vi "Dyn rolling avg.vi"(2 "N":i32=3, 4 "orig array":dbl[](array[numeric])) -> (1 "moving centered avg":dbl[](array[numeric]))   [LabVIEW 2022 SP3]
uses:
  <vilib>/Analysis/baseanly.llb/Mean (DBL).vi
  <vilib>/Analysis/NI_AALBase.lvlib
panel:
  out "Gradient Theshold":dbl
  out "Max Gradient":dbl
  out "Waveform Graph":dbl[][](graph)
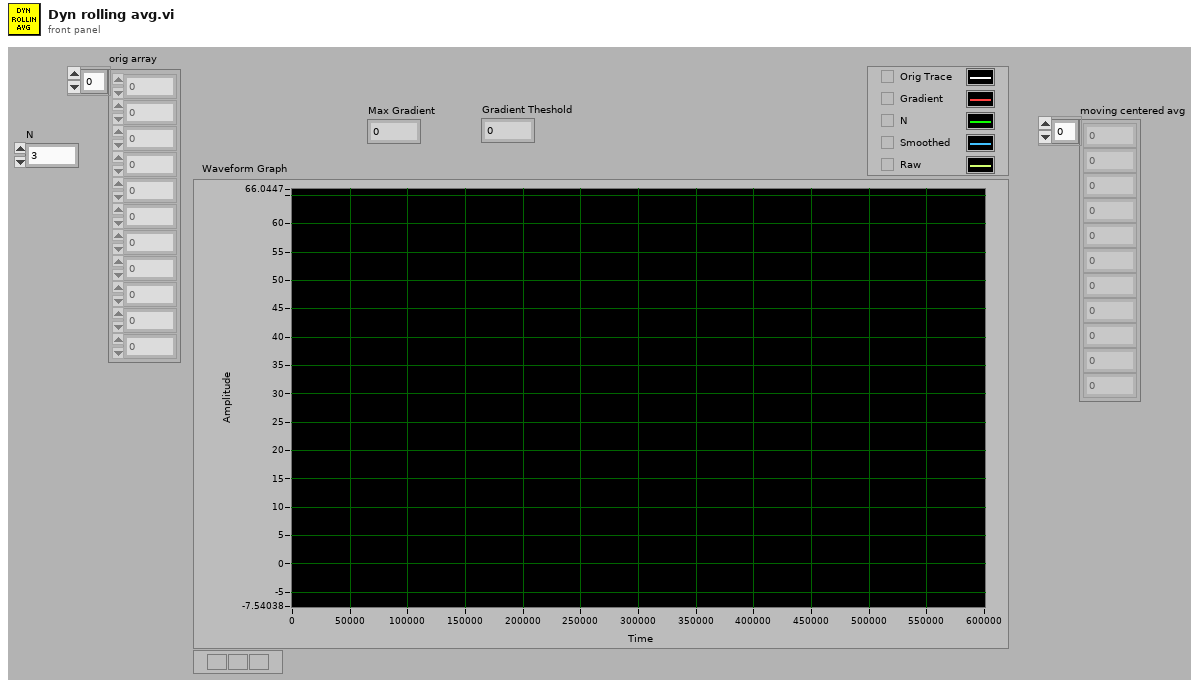
[diagram p1: front panel]
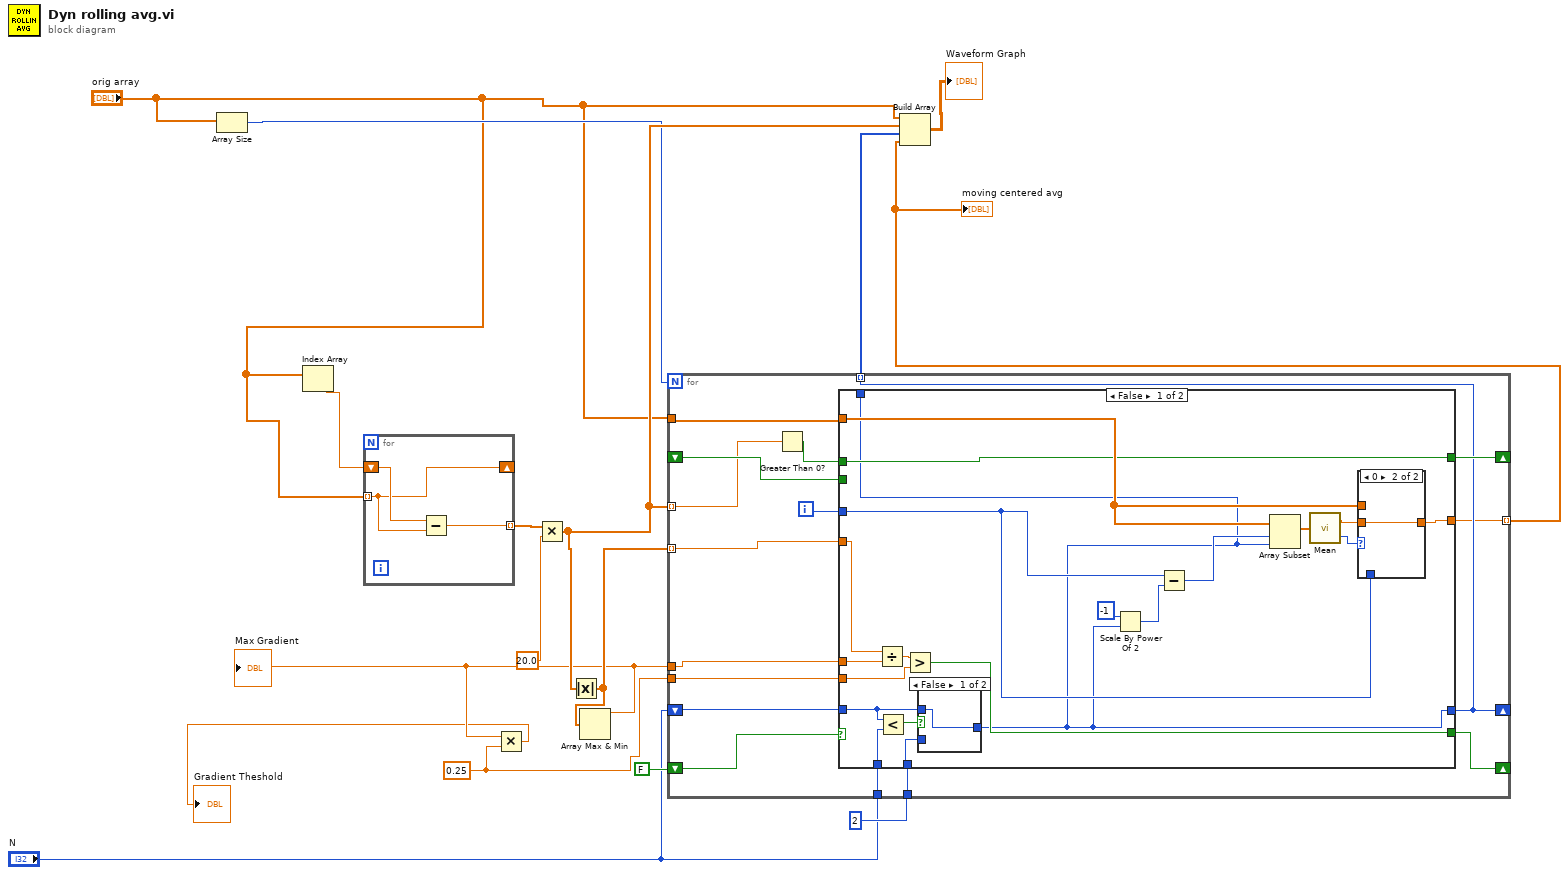
[diagram p0: block diagram]
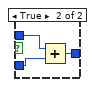
[diagram p2: hidden frame]
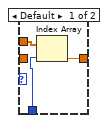
[diagram p3: hidden frame]
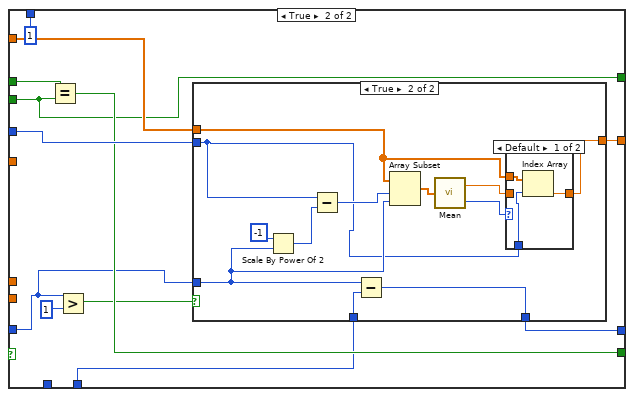
[diagram p4: hidden frame]
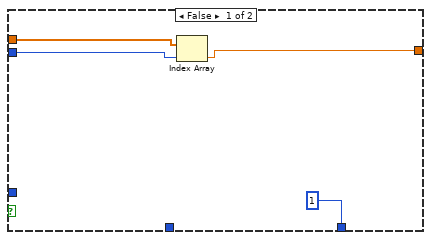
[diagram p5: hidden frame]
diagram:
  w4 = 0.25 ("y")
  n1 = Array Size(array="orig array") -> (size(s)=w7:i32)
  n2 = Index Array(array="orig array") -> (element=w15:dbl)  [unwired: 1 in]
  n3 = for {
    tunnel: "orig array" -> [w18] mode=indexing
    shift-right: [w18] -> _
    shift-left: w15 -> [w19]
    tunnel: [w17] -> w13 mode=indexing
    n4 = Subtract(x=w19, y=w18) -> (x-y=w17:dbl)
  }
  n5 = Multiply(x=w13, y=20.0) -> (x*y=w11:dbl[])
  n6 = Absolute Value(x=w11) -> (abs(x)=w12:dbl[])
  n7 = Array Max & Min(array=w12) -> (max value=w3:dbl)  [unwired: 3 out]
  "Max Gradient" <- w3
  n8 = Multiply(x=w3, y=w4) -> (x*y=→"Gradient Theshold":dbl)
  n9 = for {
    N: w7 -> [_]
    tunnel: w12 -> [w26] mode=indexing
    tunnel: w3 -> [w27]
    tunnel: "orig array" -> [w34]
    shift-right: [w31] -> _
    shift-left: _ -> [w33]
    tunnel: w11 -> [w32] mode=indexing
    shift-right: [w28] -> _
    shift-left: FALSE -> [w29]
    tunnel: [w22] -> w9 mode=indexing
    shift-right: [w22] -> _
    shift-left: "N" -> [w25]
    tunnel: 2 ("n") -> [w24]
    tunnel: "N" -> [w23]
    tunnel: w4 -> [w21]
    tunnel: [w20] -> w1 mode=indexing
    i -> [w35]
    n10 = Greater Than 0?(x=w32) -> (x > 0?=w30:bool)
    n11 = case shown="False" w29 {
      tunnel: [w55 w73] -> w20
      tunnel: w35 -> [w43 w74]
      tunnel: w34 -> [w54 w75]
      tunnel: w33 -> [_ w70]
      tunnel: [w50 w70] -> w31
      tunnel: w30 -> [w50 w72]
      tunnel: [w46 w71] -> w28
      tunnel: w27 -> [w48 _]
      tunnel: w26 -> [w47 _]
      tunnel: [w37 1 ("N")] -> _
      tunnel: w25 -> [w38 w68]
      tunnel: w24 -> [w39 w67]
      tunnel: [w37 w65] -> w22
      tunnel: w23 -> [w41 _]
      tunnel: w21 -> [w36 _]
      frame False {
        n12 = Divide(x=w47, y=w48) -> (x/y=w49:dbl)
        n13 = Less?(x=w38, y=w41) -> (x < y?=w40:bool)
        n14 = Greater?(x=w49, y=w36) -> (0:w46:bool)
        n15 = case shown="False" w40 {
          tunnel: w39 -> [_ w59]
          tunnel: w38 -> [w56 w58]
          tunnel: [w56 w57] -> w37
          frame False {
          }
          frame True {
            n16 = Add(x=w58, y=w59) -> (x+y=w57:i32)
          }
        }
        n17 = Scale By Power Of 2(n=-1, x=w37) -> (x*2^n=w44:i32)
        n18 = Subtract(x=w43, y=w44) -> (x-y=w42:i32)
        n19 = Array Subset(array=w54, index=w42, length=w37) -> (w53:dbl[])
        n20 = call-poly <vilib>:"Mean.vi"("X"=w53) -> ("mean"=w51:dbl, "error"=w52:i32)
        n21 = case shown="0" w52 {
          tunnel: [w60 w63] -> w55
          tunnel: w51 -> [_ w63]
          tunnel: w54 -> [w62 _]
          tunnel: w43 -> [w61 _]
          frame Default {
            n22 = Index Array(array=w62, index=w61) -> (element=w60:dbl)
          }
          frame 0 {
          }
        }
      }
      frame True {
        n23 = Equal?(x=w72, y=w70) -> (x = y?=w71:bool)
        n24 = Greater?(x=w68, y=1 ("n")) -> (0:w66:bool)
        n25 = case shown="True" w66 {
          tunnel: w75 -> [w79 w81]
          tunnel: w74 -> [w78 w80]
          tunnel: [w77 w82] -> w73
          tunnel: w68 -> [_ w85]
          tunnel: [1 ("n") w91] -> w65
          tunnel: w67 -> [_ w90]
          frame False {
            n26 = Index Array(array=w79, index=w78) -> (element=w77:dbl)
          }
          frame True {
            n27 = Scale By Power Of 2(n=-1, x=w85) -> (x*2^n=w88:i32)
            n28 = Subtract(x=w80, y=w88) -> (x-y=w86:i32)
            n29 = Subtract(x=w85, y=w90) -> (x-y=w91:i32)
            n30 = Array Subset(array=w81, index=w86, length=w85) -> (w87:dbl[])
            n31 = call-poly <vilib>:"Mean.vi"("X"=w87) -> ("mean"=w83:dbl, "error"=w84:i32)
            n32 = case shown="Default" w84 {
              tunnel: [w92 w95] -> w82
              tunnel: w83 -> [_ w95]
              tunnel: w81 -> [w94 _]
              tunnel: w80 -> [w93 _]
              frame Default {
                n33 = Index Array(array=w94, index=w93) -> (element=w92:dbl)
              }
              frame 0 {
              }
            }
          }
        }
      }
    }
  }
  "moving centered avg" <- w1
  n34 = Build Array("orig array", w11, w9, w1) -> (→"Waveform Graph":dbl[][])
